vi "Mod Queue - Destroy.vi"(8 "error in":errorcluster) -> (0 "error out":errorcluster)   [LabVIEW 2024]
uses:
  General Type Defs/FGV States.ctl
  General Type Defs/General Type Definitions.lvlib
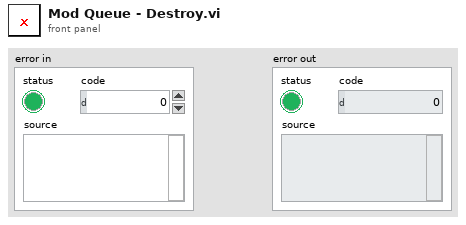
[diagram p1: front panel]
types:
  T1 = typedef "General Type Definitions.lvlib/FGV States.ctl" = enum16{"Create", "Get", "Destroy"}
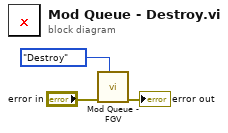
[diagram p0: block diagram]
diagram:
  n1 = call "Mod Queue - FGV.vi"("FGV States"=FGV_States."Destroy", "error in"="error in") -> ("error out"=→"error out":errorcluster)  [unwired: 8 in, 1 out]
